vi "PH_Beckhoff.handle Digital Outputs.vi"(0 "i ref in":refnum<vi>, 1 "Old Values":T1, 2 "Current Digital Outputs":bool[](array[boolean]), 3 "Quality":bool, 5 "error in":errorcluster) -> (14 "i ref out":refnum<vi>, 17 "#s of changed digital Outputs":i32[](array[numeric]), 19 "error out":errorcluster)   [LabVIEW 2014, in "PH_Beckhoff.lvlib"]
doc: "This VI handles the incoming information about digital inputs: if value or quality changed, these are set to own attributes and the scaled information is published via DIM."
uses:
  PH_Beckhoff.lvlib
  PH_Beckhoff.Values.ctl
  PH_Beckhoff.Sonderklemmen Inputs.ctl
  PH_Beckhoff.Analog Inputs.ctl
  PH_Beckhoff.Scaling Type.ctl
  PH_Beckhoff.Analog Outputs.ctl
  PH_Beckhoff.Digital Inputs.ctl
  PH_Beckhoff.Digital Outputs.ctl
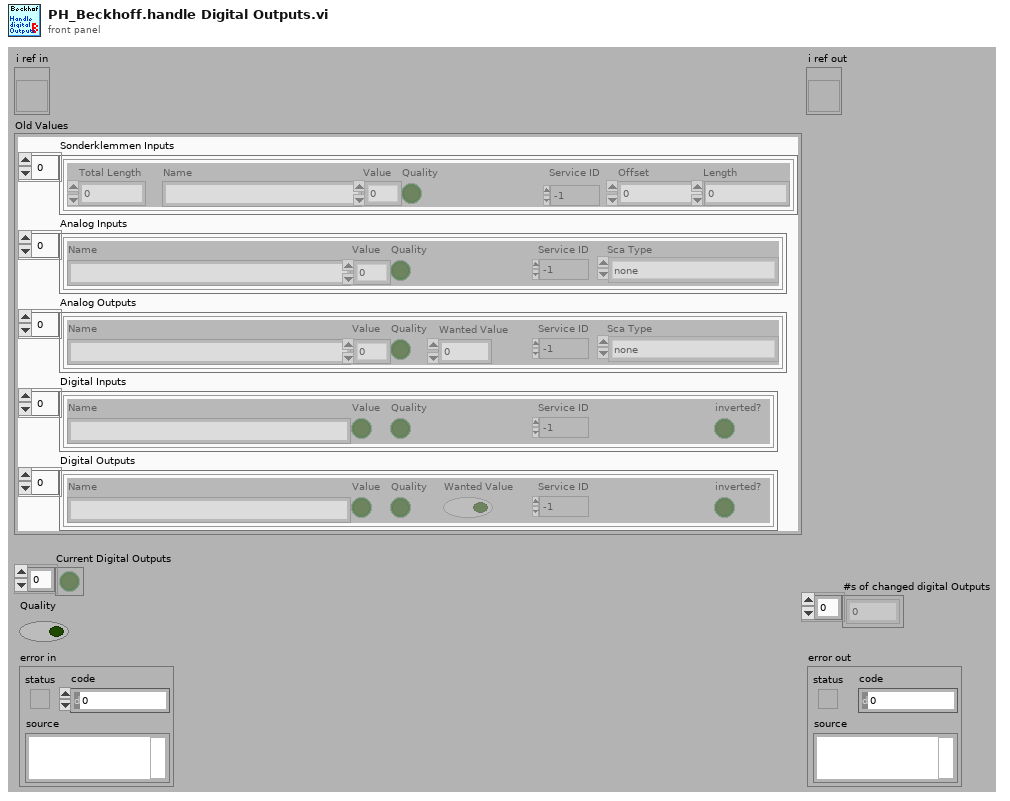
[diagram p1: front panel]
types:
  T1 = typedef "PH_Beckhoff.lvlib/PH_Beckhoff.Values.ctl" = cluster{"Sonderklemmen Inputs":T2, "Analog Inputs":T3, "Analog Outputs":T5, "Digital Inputs":T6, "Digital Outputs":T7}
  T2 = typedef "PH_Beckhoff.lvlib/PH_Beckhoff.Sonderklemmen Inputs.ctl" = cluster{"Total Length":u32, "Name":string, "Value":u64, "Quality":bool, "Service ID":i32, "Offset":u32, "Length":u32}[]
  T3 = typedef "PH_Beckhoff.lvlib/PH_Beckhoff.Analog Inputs.ctl" = cluster{"Name":string, "Value":u32, "Quality":bool, "Service ID":i32, "Sca Type":T4}[]
  T4 = typedef "PH_Beckhoff.lvlib/PH_Beckhoff.Scaling Type.ctl" = enum16{"none", "0 ... 15 Bit -> 0 ... 5", "0 ... 15 Bit -> 0 ... 10", "0 ... 15 Bit -> 0 ... 25", "0 ... 15 Bit -> 4 ... 20", "0 ... 15 Bit -> 0 ... 1", "0 ... 15 Bit -> 0 ... 20000", "0 ... 15 Bit -> 0 ... 24000"}
  T5 = typedef "PH_Beckhoff.lvlib/PH_Beckhoff.Analog Outputs.ctl" = cluster{"Name":string, "Value":u32, "Quality":bool, "Wanted Value":u32, "Service ID":i32, "Sca Type":T4}[]
  T6 = typedef "PH_Beckhoff.lvlib/PH_Beckhoff.Digital Inputs.ctl" = cluster{"Name":string, "Value":bool, "Quality":bool, "Service ID":i32, "inverted?":bool}[]
  T7 = typedef "PH_Beckhoff.lvlib/PH_Beckhoff.Digital Outputs.ctl" = cluster{"Name":string, "Value":bool, "Quality":bool, "Wanted Value":bool, "Service ID":i32, "inverted?":bool}[]
  T8 = typedef "PH_Beckhoff.lvlib/PH_Beckhoff.i attribute.ctl" = cluster{"GUI Refs":T9, "operation?":bool, "Default Prdc Interval":i32, "Connection":T10, "AMS Net ID":T11, "Klemmencluster: # of":T12, "Values":T1, "IP":string, "Description":string, "configured?":bool, "Change Manager":cluster{"Detemination wanted?":bool, "Values changed at":cluster{"Sonderklemmen Inputs":i32[], "Analog Inputs":i32[], "Analog Outputs":i32[], "Digital Inputs":i32[], "Digital Outputs":i32[]}}, "Difference to handle an analog input as change":u32}
  T9 = typedef "PH_Beckhoff.lvlib/PH_Beckhoff.GUI Refs.ctl" = cluster{"ADS Error":refnum<vi>, "Values":refnum<vi>, "configured?":refnum<vi>, "Connection":refnum<vi>, "IP":refnum<vi>, "Prdc Int [ms]":refnum<vi>}
  T10 = typedef "PH_Beckhoff.lvlib/PH_Beckhoff.Connectivity.ctl" = cluster{"DLL?":bool, "Port?":bool, "Client?":bool, "Ping?":bool, "unsuccessful Pings":u32}
  T11 = typedef "Beckhoff - Driver np.lvlib/Beckhoff Access.ctl" = cluster{"DLL path":path, "AMS Net ID":cluster{"1st # of IP":u8, "2nd # of IP":u8, "3rd # of IP":u8, "4th # of IP":u8, "In Port":u8, "Out Port":u8}}
  T12 = typedef "Beckhoff - Driver np.lvlib/Klemmendeclarer.ctl" = cluster{"Offset due to Sonderklemms":u32, "analog Inputs":u32, "analog Outputs":u32, "digital Input Bits":u32, "digital Output Bits":u32}
  T13 = cluster{"Name":string, "Value":bool, "Quality":bool, "Wanted Value":bool, "Service ID":i32, "inverted?":bool}
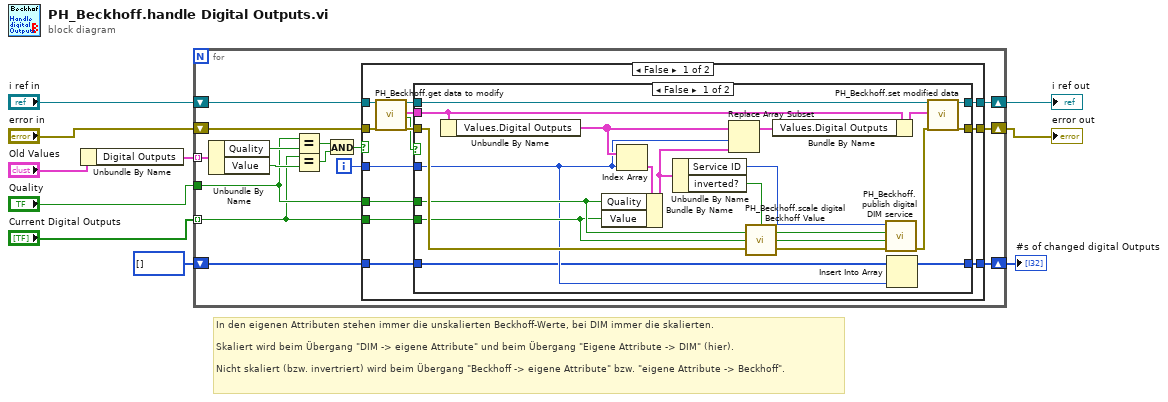
[diagram p0: block diagram]
diagram:
  # "In den eigenen Attributen stehen immer die unskalierten Beckhoff-Werte, bei DIM immer die skalierten.\n\nSkaliert wird beim Übergang \"DIM -> eigene Attribute\" und beim Übergang \"Eigene Attribute -> DIM\" (hier).\n\nNicht skaliert (bzw. invertriert) wird beim Übergang \"Beckhoff -> eigene Attribute\" bzw. \"eigene Attribute -> Beckhoff\"."
  n1 = Unbundle By Name("Old Values") -> ("Digital Outputs"=w10:T7)
  n2 = for {
    tunnel: w10 -> [w25] mode=indexing
    tunnel: "Quality" -> [w14]
    tunnel: "Current Digital Outputs" -> [w13] mode=indexing
    shift-right: [w18] -> w7
    shift-left: "error in" -> [w19]
    shift-right: [w16] -> w6
    shift-left: "i ref in" -> [w17]
    shift-right: [w12] -> w2
    shift-left: i32[] [] -> [w11]
    i -> [w15]
    n3 = Unbundle By Name(w25) -> ("Quality"=w23:bool, "Value"=w24:bool)
    n4 = Equal?(x=w14, y=w23) -> (x = y?=w22:bool)
    n5 = Equal?(x=w13, y=w24) -> (x = y?=w21:bool)
    n6 = And(x=w22, y=w21) -> (x .and. y?=w20:bool)
    n7 = case shown="False" w20 {
      tunnel: w19 -> [w38 w63]
      tunnel: [w36 w63] -> w18
      tunnel: w17 -> [w35 w62]
      tunnel: [w33 w62] -> w16
      tunnel: w15 -> [w30 _]
      tunnel: w14 -> [w29 _]
      tunnel: w13 -> [w28 _]
      tunnel: [w27 w61] -> w12
      tunnel: w11 -> [w26 w61]
      frame False {
        n8 = call "PH_Beckhoff.get data to modify.vi"("i ref in"=w35, "error in (no error)"=w38) -> ("i ref out"=w34:refnum<vi>, "i attribute"=w31:T8, "timed out"=w32:bool, "error out"=w37:errorcluster)  [unwired: 14 in]
        n9 = case shown="False" w32 {
          tunnel: w37 -> [w47 w59]
          tunnel: [w57 w59] -> w36
          tunnel: w34 -> [w56 w60]
          tunnel: [w55 w60] -> w33
          tunnel: w31 -> [w53 _]
          tunnel: w30 -> [w40 _]
          tunnel: w29 -> [w45 _]
          tunnel: w28 -> [w44 _]
          tunnel: [w41 w58] -> w27
          tunnel: w26 -> [w39 w58]
          frame False {
            n10 = Unbundle By Name(w53) -> ("Values.Digital Outputs"=w51:T7)
            n11 = Index Array(array=w51, index=w40) -> (element=w50:T13)
            n12 = Bundle By Name(cluster=w50, "Quality"=w45, "Value"=w44) -> (w46:T13)
            n13 = Unbundle By Name(w46) -> ("Service ID"=w48:i32, "inverted?"=w42:bool)
            n14 = Replace Array Subset(array=w51, new element=w46, index=w40) -> (w52:T7)
            n15 = call "PH_Beckhoff.scale digital Beckhoff Value.vi"("Beckhoff value"=w44, "inverted?"=w42) -> ("DIM value"=w43:bool)
            n16 = Bundle By Name(cluster=w53, "Values.Digital Outputs"=w52) -> (w54:T8)
            n17 = call "PH_Beckhoff.publish digital DIM service.vi"("error in"=w47, "Value"=w43, "Quality ok?"=w45, "Service ID"=w48) -> ("error out"=w49:errorcluster)  [unwired: 4 in]
            n18 = Insert Into Array(array=w39, new element=w40) -> (w41:i32[])  [unwired: 1 in]
            n19 = call "PH_Beckhoff.set modified data.vi"("i ref in"=w56, "i attribute"=w54, "error in (no error)"=w49) -> ("i ref out"=w55:refnum<vi>, "error out"=w57:errorcluster)  [unwired: 15 in]
          }
          frame True {
          }
        }
      }
      frame True {
      }
    }
  }
  "i ref out" <- w6
  "error out" <- w7
  "#s of changed digital Outputs" <- w2
